vi "HCalculator (SubVI).vi"(8 "Turns of Coil":dbl=6.0, 9 "Rokoski (V(mV)/I(A))":dbl=20.0, 10 "H calculator":bool, 11 "Vpp in":dbl) -> (2 "Vpp out":dbl, 3 "Current (A)":dbl)   [LabVIEW 2015]
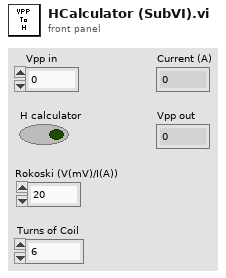
[diagram p1: front panel]
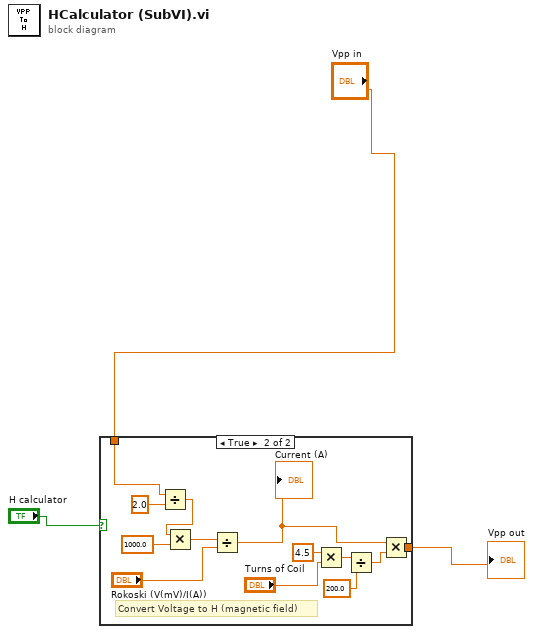
[diagram p0: block diagram]
diagram:
  n1 = case shown="True" "H calculator" {
    tunnel: "Vpp in" -> [w4 w7]
    tunnel: [w4 w8] -> w3
    frame False {
    }
    frame True {
      # "Convert Voltage to H (magnetic field)"
      n2 = Divide(x=w7, y=2.0) -> (x/y=w5:dbl)
      n3 = Multiply(x=w5, y=1000.0) -> (x*y=w16:dbl)
      n4 = Divide(x=w16, y="Rokoski (V(mV)/I(A))") -> (x/y=w10:dbl)
      "Current (A)" <- w10
      n5 = Multiply(x=4.5, y="Turns of Coil") -> (x*y=w12:dbl)
      n6 = Divide(x=w12, y=200.0) -> (x/y=w9:dbl)
      n7 = Multiply(x=w10, y=w9) -> (x*y=w8:dbl)
    }
  }
  "Vpp out" <- w3
